vi "Equip-Get AI Channels (String).vi"(0 "Path":path, 7 "Inputs":string[](array[string]), 11 "error in (no error)":errorcluster) -> (8 "AI Channels":i32[](array[numeric]), 15 "error out":errorcluster)   [LabVIEW 2020]
uses:
  <vilib>/Utility/config.llb/Read Key (I32).vi
  <vilib>/Utility/config.llb/NI_LVConfig.lvlib
panel:
  in  "section":string="Connections"
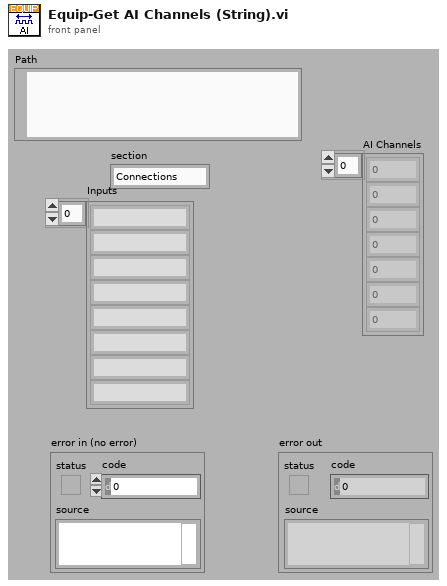
[diagram p1: front panel]
types:
  T1 = typedef "NI_LVConfig.lvlib/Config Data RefNum.ctl" = refnum<k1>
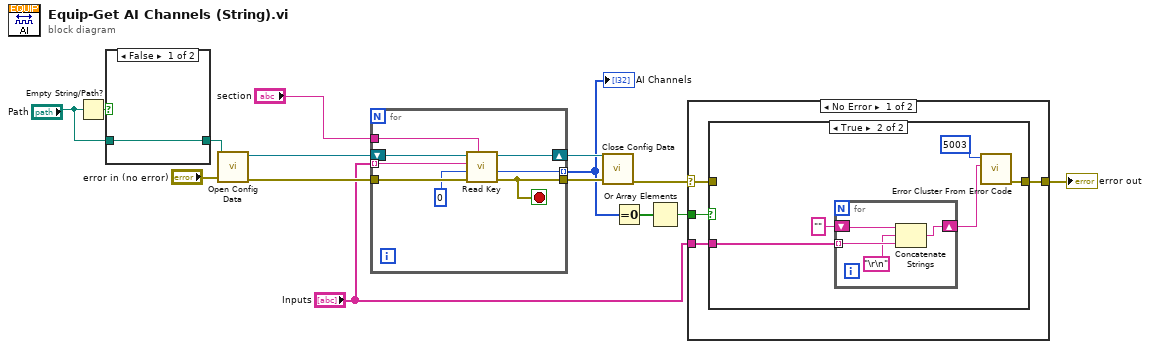
[diagram p0: block diagram]
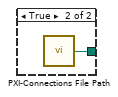
[diagram p2: hidden frame]
diagram:
  n1 = Empty String/Path?(string/path="Path") -> (empty?=w4:bool)
  n2 = case shown="False" w4 {
    tunnel: [w16 w17] -> w2
    tunnel: "Path" -> [w16 _]
    frame False {
    }
    frame True {
      n3 = call "PXI-Connections File Path.vi"() -> ("Path"=w17:path)  [unwired: 1 in]
    }
  }
  n4 = call <vilib>:"Open Config Data.vi"("error in (no error)"="error in (no error)", "configuration file path"=w2) -> ("error out"=w7:errorcluster, "refnum"=w6:T1)  [unwired: 7 in, 1 out]
  n5 = for {
    tunnel: "Inputs" -> [w18] mode=indexing
    tunnel: [w22] -> w12 mode=indexing
    tunnel: "section" -> [w20]
    tunnel: w7 -> [w25]
    tunnel: [w19] -> w14
    shift-right: [w21] -> w13
    shift-left: w6 -> [w24]
    stop <- w19 stop-if-true
    n6 = call-poly <vilib>:"Read Key.vi"("section"=w20, "error in (no error)"=w25, "default value"=0, "key"=w18, "refnum"=w24) -> ("error out"=w19:errorcluster, "value"=w22:i32, "refnum out"=w21:T1)  [unwired: 3 in, 1 out]
  }
  "AI Channels" <- w12
  n7 = call <vilib>:"Close Config Data.vi"("error in (no error)"=w14, "refnum"=w13) -> ("error out"=w8:errorcluster)  [unwired: 8 in, 1 out]
  n8 = Equal To 0?(x=w12) -> (x = 0?=w11:bool[])
  n9 = Or Array Elements(Boolean array=w11) -> (logical OR=w10:bool)
  n10 = case shown="No Error" w8 {
    selector: w8 -> [w27 w40]
    tunnel: w10 -> [w29 _]
    tunnel: [w28 w40] -> w9
    tunnel: "Inputs" -> [w26 _]
    frame No Error {
      n11 = case shown="True" w29 {
        tunnel: w27 -> [w30 _]
        tunnel: [w30 w35] -> w28
        tunnel: w26 -> [_ w33]
        frame False {
        }
        frame True {
          n12 = for {
            tunnel: w33 -> [w38] mode=indexing
            shift-right: [w39] -> w32
            shift-left: "" -> [w36]
            n13 = Concatenate Strings(w36, "\r\n", w38) -> (w39:string)
          }
          n14 = call <vilib>:"Error Cluster From Error Code.vi"("error message (\"\")"=w32, "error code (0)"=5003) -> ("error out"=w35:errorcluster)  [unwired: 7 in]
        }
      }
    }
    frame Error {
    }
  }
  "error out" <- w9
